vi "GVUTC_ECD.vi"() -> ()   [LabVIEW 2017]
panel:
  out "GV UTC":dbl
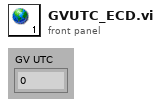
[diagram p1: front panel]
diagram:
